vi "Main.vi"(8 "error in":errorcluster, 11 "WaveGenerator in":refnum<class "WaveGenerator.lvclass">) -> (0 "error out":errorcluster, 3 "WaveGenerator out":refnum<class "WaveGenerator.lvclass">)   [LabVIEW 2017, in "WaveGenerator.lvclass"]
doc: "The Queued Message Handler of a Worker."
uses:
  WaveGenerator.lvclass
  Initialization Data.ctl
  <vilib>/addons/_Workers/Library/Classes/Callback Message/Callback Message.lvclass
  <vilib>/addons/_Workers/Library/Classes/Worker/Worker.lvclass
  <vilib>/addons/_Workers/Library/Classes/Worker/Read Alias.vi
  <vilib>/addons/_Workers/Library/Case Label.ctl
  <vilib>/addons/_Workers/Library/Workers.lvlib
  <vilib>/addons/_Workers/Library/Classes/Message Queue/Message Queue.lvclass
  <vilib>/addons/_Workers/Library/Classes/Message/Message.lvclass
  <vilib>/addons/_Workers/Library/Classes/Message/Enqueue Message to Self v2.vi
  48f7c94d-1f04-4e88-be23-9017f90e960e.vi
  <vilib>/addons/_Workers/Library/Classes/Message/Enqueue Message to Queue - Silent Mode.vi
  <vilib>/addons/_Workers/Library/Classes/Message/Enqueue Message to Self v2 - Silent Mode.vi
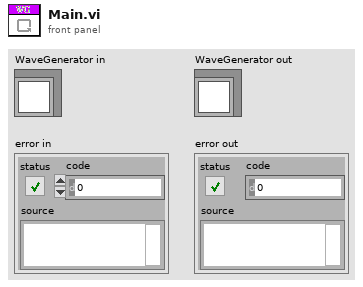
[diagram p1: front panel]
types:
  T1 = typedef "WaveGenerator.lvclass/Initialization Data.ctl" = cluster{"String":string}
  T2 = typedef "Workers.lvlib/Case Label.ctl" = string
  T3 = cluster{"Message Queue out":refnum<class "Message Queue.lvclass">, "Case Label":T2}
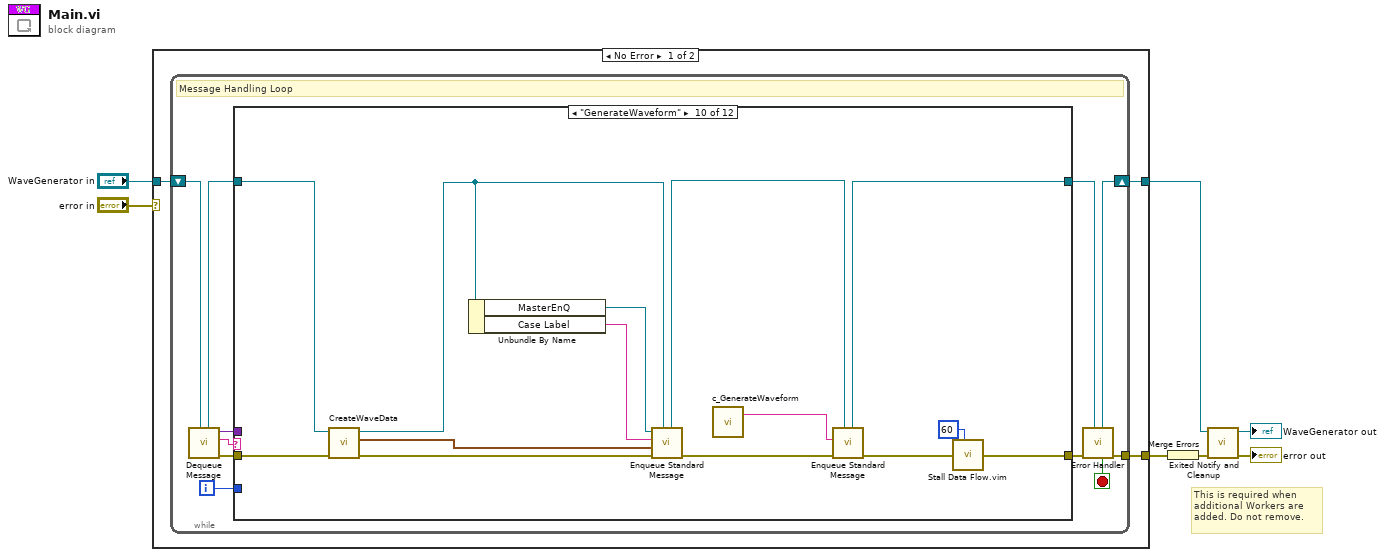
[diagram p0: block diagram]
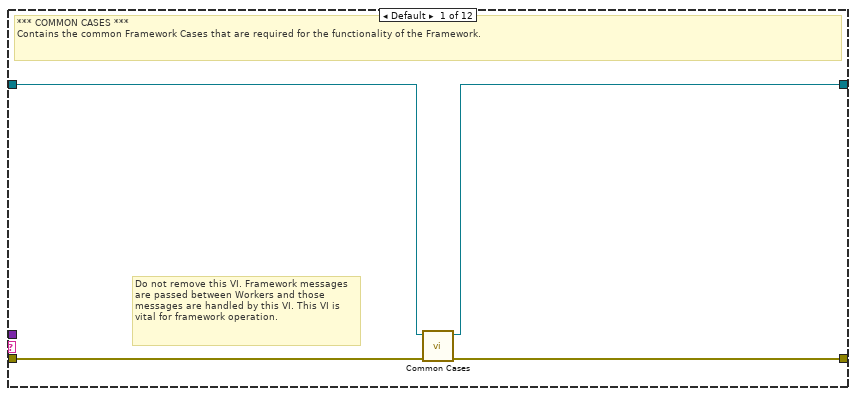
[diagram p2: hidden frame]
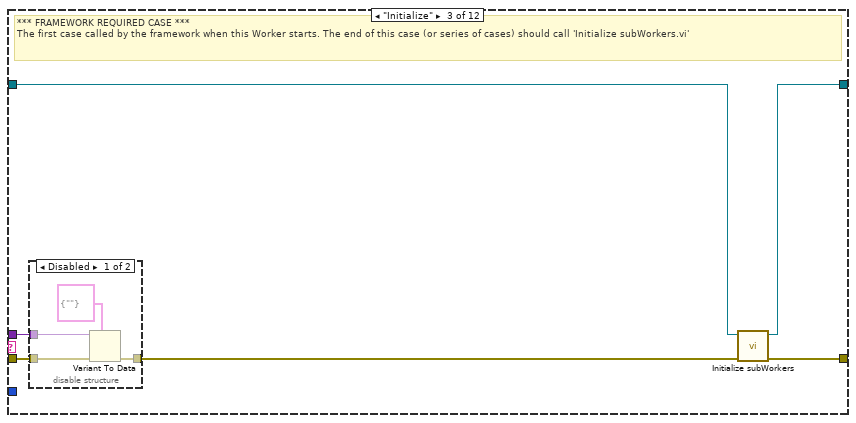
[diagram p4: hidden frame]
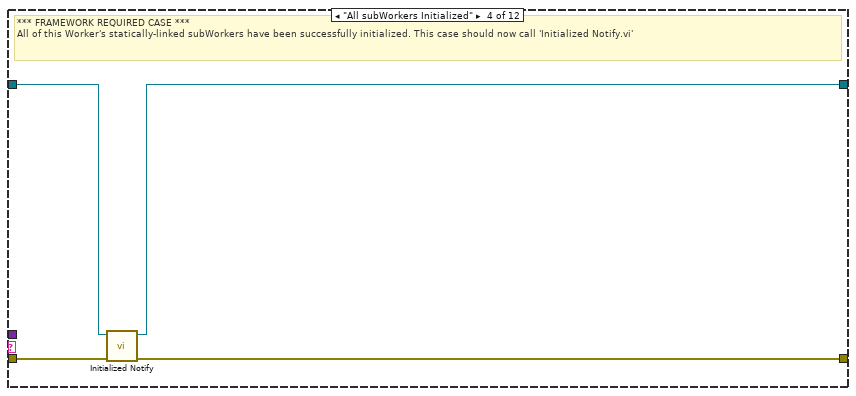
[diagram p6: hidden frame]
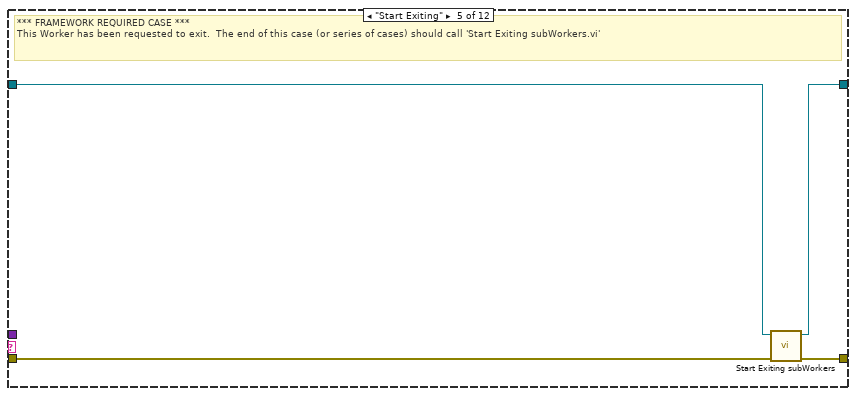
[diagram p7: hidden frame]
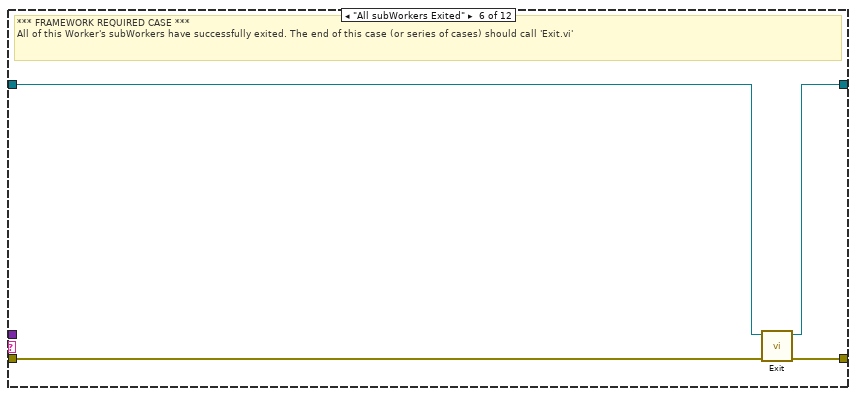
[diagram p8: hidden frame]
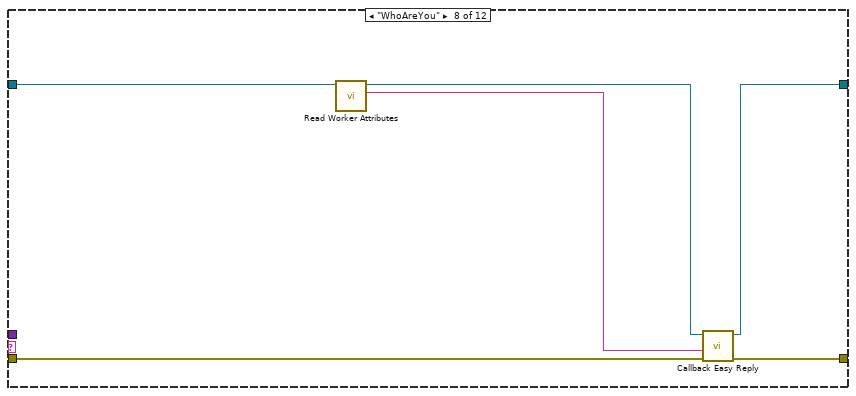
[diagram p10: hidden frame]
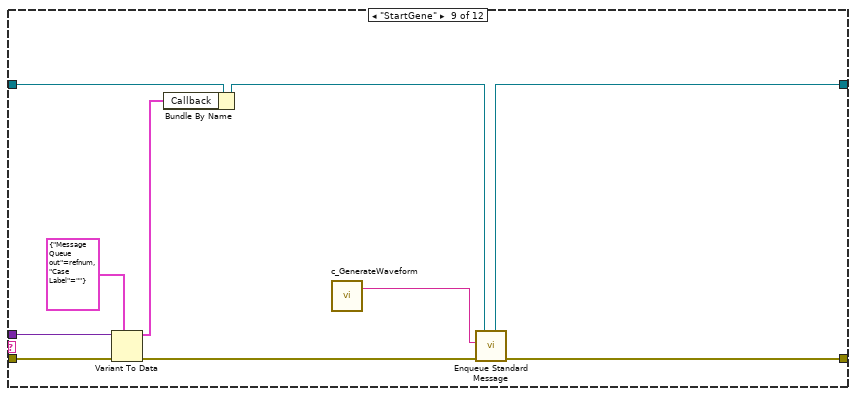
[diagram p11: hidden frame]
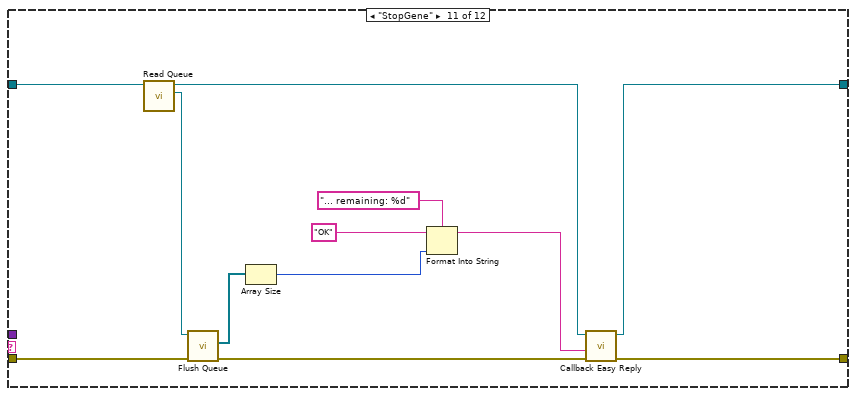
[diagram p12: hidden frame]
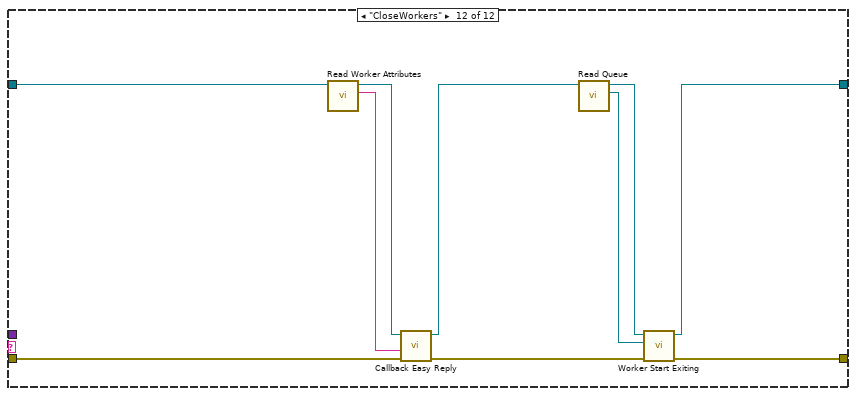
[diagram p13: hidden frame]
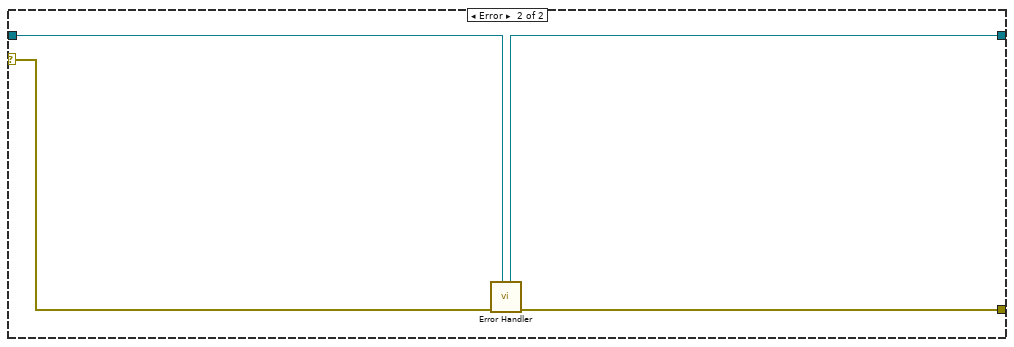
[diagram p14: hidden frame]
diagram:
  # "This is required when additional Workers are added. Do not remove."
  n1 = case shown="No Error" "error in" {
    tunnel: "WaveGenerator in" -> [w8 w106]
    tunnel: [w10 w107] -> w6
    tunnel: [w9 w105] -> w7
    selector: "error in" -> [_ w108]
    frame No Error {
      n2 = while {
        shift-right: [w19] -> w9
        shift-left: w8 -> [w21]
        tunnel: [w20] -> w10
        i -> [w11]
        stop <- w12 stop-if-true
        # "Message Handling Loop"
        n3 = call-dynamic "Dequeue Message.vi"("Worker"=w21) -> ("error out"=w18:errorcluster, "Case out"=w13:string, "Data out"=w14:variant, "Worker out"=w16:refnum<class "WaveGenerator.lvclass">)  [unwired: 6 in, 1 out]
        n4 = case "Worker MHL Case Structure (DO NOT CHANGE LABEL NAME)" shown="\"GenerateWaveform\"" w13 {
          tunnel: w18 -> [w25 w26 w31 w42 w43 w50 w51 w58 w68 w82 w92 w104]
          tunnel: [w24 w26 w33 w41 w46 w49 w51 w57 w62 w70 w90 w103] -> w17
          tunnel: w16 -> [w23 w27 w30 w40 w44 w48 w52 w56 w67 w79 w94 w98]
          tunnel: [w22 w27 w32 w39 w45 w47 w52 w55 w60 w72 w88 w102] -> w15
          tunnel: w14 -> [_ _ w28 _ _ _ _ _ w65 _ _ _]
          tunnel: w11 -> [_ _ _ _ _ _ _ _ _ _ _ _]
          frame Default {
            # "Do not remove this VI. Framework messages are passed between Workers and those messages are handled by this VI. This VI is vital for framework operation."
            # "*** COMMON CASES ***\nContains the common Framework Cases that are required for the functionality of the Framework."
            n5 = call-dynamic "Common Cases.vi"("error in"=w25, "Worker in"=w23) -> ("error out"=w24:errorcluster, "Worker out"=w22:refnum<class "WaveGenerator.lvclass">)  [unwired: 8 in]
          }
          frame "------ FRAMEWORK REQUIRED CASES ------" {
            # "Start of Framework Required Cases"
          }
          frame "Initialize" {
            # "*** FRAMEWORK REQUIRED CASE ***\nThe first case called by the framework when this Worker starts. The end of this case (or series of cases) should call 'Initialize subWorkers.vi'"
            n6 = disable-structure shown="Disabled" {
              disable-tunnel: w31 -> [w37 w38]
              disable-tunnel: [w36 w38] -> w29
              disable-tunnel: w28 -> [w34 _]
              frame Disabled {
                n7 = Variant To Data(error in=w37, type=T1 {"String"=""} ("Cluster"), Variant=w34) -> (error out=w36:errorcluster)  [unwired: 1 out]
              }
              frame Enabled {
              }
            }
            n8 = call-dynamic "Initialize subWorkers.vi"("error in"=w29, "Worker"=w30) -> ("error out"=w33:errorcluster, "dup Worker out"=w32:refnum<class "WaveGenerator.lvclass">)  [unwired: 8 in]
          }
          frame "All subWorkers Initialized" {
            # "*** FRAMEWORK REQUIRED CASE ***\nAll of this Worker's statically-linked subWorkers have been successfully initialized. This case should now call 'Initialized Notify.vi'"
            n9 = call-dynamic "Initialized Notify.vi"("error in"=w42, "Worker"=w40) -> ("error out"=w41:errorcluster, "dup Worker out"=w39:refnum<class "WaveGenerator.lvclass">)  [unwired: 8 in]
          }
          frame "Start Exiting" {
            # "*** FRAMEWORK REQUIRED CASE ***\nThis Worker has been requested to exit.  The end of this case (or series of cases) should call 'Start Exiting subWorkers.vi'"
            n10 = call-dynamic "Start Exiting subWorkers.vi"("error_in"=w43, "Worker"=w44) -> ("error out"=w46:errorcluster, "dup Worker out"=w45:refnum<class "WaveGenerator.lvclass">)  [unwired: 8 in]
          }
          frame "All subWorkers Exited" {
            # "*** FRAMEWORK REQUIRED CASE ***\nAll of this Worker's subWorkers have successfully exited. The end of this case (or series of cases) should call 'Exit.vi'"
            n11 = call-dynamic "Exit.vi"("error_in"=w50, "Worker"=w48) -> ("error out"=w49:errorcluster, "dup Worker out"=w47:refnum<class "WaveGenerator.lvclass">)  [unwired: 8 in]
          }
          frame "-----------------------------------------------" {
            # "End of Framework Required Cases"
          }
          frame "WhoAreYou" {
            n12 = call-poly <vilib>:"Read Worker Attributes.vi"("Worker"=w56) -> ("Alias out"=w53:string, "dup Worker out"=w54:refnum<class "WaveGenerator.lvclass">)  [unwired: 9 in]
            n13 = call <vilib>:"Callback Easy Reply.vi"("error in"=w58, "Data"=w53, "Worker"=w54) -> ("error out"=w57:errorcluster, "dup Worker out"=w55:refnum<class "WaveGenerator.lvclass">)  [unwired: 7 in]
          }
          frame "StartGene" {
            n14 = Variant To Data(error in=w68, type=T3 {"Message Queue out"=refnum, "Case Label"=""} ("output cluster"), Variant=w65) -> (data=w63:T3, error out=w66:errorcluster)
            n15 = Bundle By Name(cluster=w67, "Callback"=w63) -> (w61:refnum<class "WaveGenerator.lvclass">)
            n16 = call "c_GenerateWaveform.vi"() -> ("Case Label"=w59:T2)  [unwired: 1 in]
            n17 = call-poly <vilib>:"Enqueue Standard Message.vi"("Worker"=w61, "error in"=w66, "Case Label"=w59) -> ("error out"=w62:errorcluster, "dup Worker out"=w60:refnum<class "WaveGenerator.lvclass">)  [unwired: 7 in]
          }
          frame "GenerateWaveform" {
            n18 = call-dynamic "CreateWaveData.vi"("error in (no error)"=w82, "WaveGenerator in"=w79) -> ("error out"=w81:errorcluster, "signal out"=w78:waveform(dbl), "WaveGenerator out"=w77:refnum<class "WaveGenerator.lvclass">)  [unwired: 7 in]
            n19 = Unbundle By Name(w77) -> ("MasterEnQ"=w76:refnum<class "Message Queue.lvclass">, "Case Label"=w75:T2)
            n20 = call-poly <vilib>:"Enqueue Standard Message.vi"("Worker"=w77, "error in"=w81, "Data"=w78, "Case Label"=w75, "Message Queue"=w76) -> ("error out"=w80:errorcluster, "dup Worker out"=w73:refnum<class "WaveGenerator.lvclass">)  [unwired: 4 in, 1 out]
            n21 = call "c_GenerateWaveform.vi"() -> ("Case Label"=w71:T2)  [unwired: 1 in]
            n22 = call-poly <vilib>:"Enqueue Standard Message.vi"("Worker"=w73, "error in"=w80, "Case Label"=w71) -> ("error out"=w74:errorcluster, "dup Worker out"=w72:refnum<class "WaveGenerator.lvclass">)  [unwired: 7 in]
            n23 = call "Stall Data Flow.vim"("value in"=w74, "milliseconds to wait"=u32 60) -> ("value out"=w70:errorcluster)  [unwired: 1 out]
          }
          frame "StopGene" {
            n24 = call <vilib>:"Read Queue.vi"("Worker"=w94) -> ("Message Queue out"=w93:refnum<class "Message Queue.lvclass">, "dup Worker out"=w89:refnum<class "WaveGenerator.lvclass">)  [unwired: 9 in]
            n25 = call <vilib>:"Flush Queue.vi"("error in (no error)"=w92, "Message Queue"=w93) -> ("error out"=w91:errorcluster, "remaining elements"=w86:refnum<class "Message.lvclass">[])  [unwired: 7 in, 1 out]
            n26 = Array Size(array=w86) -> (size(s)=w83:i32)
            n27 = Format Into String(format string="... remaining: %d", initial string="OK", w83) -> (resulting string=w85:string)  [unwired: 1 in, 1 out]
            n28 = call <vilib>:"Callback Easy Reply.vi"("error in"=w91, "Data"=w85, "Worker"=w89) -> ("error out"=w90:errorcluster, "dup Worker out"=w88:refnum<class "WaveGenerator.lvclass">)  [unwired: 7 in]
          }
          frame "CloseWorkers" {
            n29 = call-poly <vilib>:"Read Worker Attributes.vi"("Worker"=w98) -> ("Alias out"=w95:string, "dup Worker out"=w96:refnum<class "WaveGenerator.lvclass">)  [unwired: 9 in]
            n30 = call <vilib>:"Callback Easy Reply.vi"("error in"=w104, "Data"=w95, "Worker"=w96) -> ("error out"=w99:errorcluster, "dup Worker out"=w97:refnum<class "WaveGenerator.lvclass">)  [unwired: 7 in]
            n31 = call <vilib>:"Read Queue.vi"("Worker"=w97) -> ("Message Queue out"=w100:refnum<class "Message Queue.lvclass">, "dup Worker out"=w101:refnum<class "WaveGenerator.lvclass">)  [unwired: 9 in]
            n32 = call-dynamic "Worker Start Exiting.vi"("error_in"=w99, "Message Queue"=w100, "Worker"=w101) -> ("error out"=w103:errorcluster, "dup Worker out"=w102:refnum<class "WaveGenerator.lvclass">)  [unwired: 7 in]
          }
        }
        n33 = call-dynamic "Error Handler.vi"("Worker"=w15, "error_in"=w17) -> ("error out"=w20:errorcluster, "Stop Loop"=w12:bool, "Worker out"=w19:refnum<class "WaveGenerator.lvclass">)  [unwired: 7 in]
      }
    }
    frame Error {
      n34 = call-dynamic "Error Handler.vi"("Worker"=w106, "error_in"=w108) -> ("error out"=w107:errorcluster, "Worker out"=w105:refnum<class "WaveGenerator.lvclass">)  [unwired: 7 in, 1 out]
    }
  }
  n35 = Merge Errors(w6) -> (w3:errorcluster)
  n36 = call-dynamic "Exited Notify and Cleanup.vi"("error_in"=w3, "Worker"=w7) -> ("error out"=→"error out":errorcluster, "dup Worker out"=→"WaveGenerator out":refnum<class "WaveGenerator.lvclass">)  [unwired: 8 in]
